vi "Do.vi"(8 "error in (no error)":errorcluster, 10 "Actor in":refnum<class "Actor.lvclass">, 11 "Execute Channel Msg":refnum<class "Execute Channel Msg.lvclass">) -> (0 "error out":errorcluster, 2 "Actor out":refnum<class "Actor.lvclass">)   [LabVIEW 2014, in "Generic Data Acquisition.lvlib" / "National Instrument USB-6501.lvlib" / "Execute Channel Msg.lvclass"]
doc: "This VI delivers the message to the actor by calling the appropriate method(s) on the actor."
uses:
  Execute Channel Msg.lvclass
  <vilib>/ActorFramework/Actor/Actor.lvclass
  National Instrument USB-6501/National Instrument USB-6501.lvclass
  Execute Channel Msg.lvclass/Execute Channel Msg.ctl
  <resource>/objmgr/daqmx.rc
panel:
  out "IsGlobal":bool
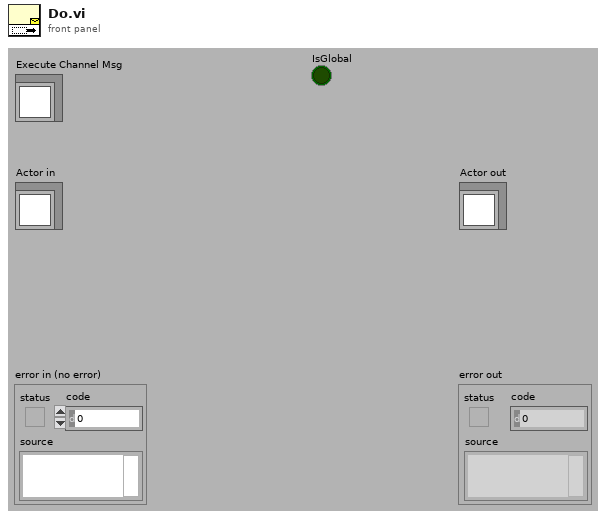
[diagram p1: front panel]
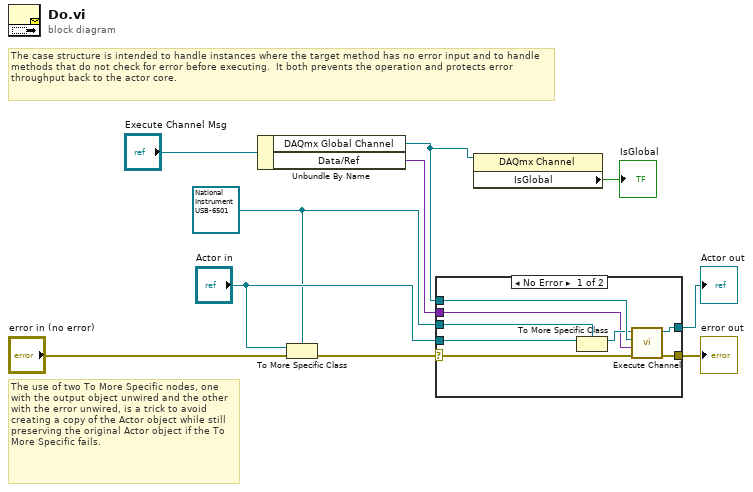
[diagram p0: block diagram]
diagram:
  w4 = refnum<class "National Instrument USB-6501.lvclass"> refnum ("Actor in")
  # "The use of two To More Specific nodes, one with the output object unwired and the other with the error unwired, is a trick to avoid creating a copy of the Actor object while still preserving the original Actor object if the To More Specific fails."
  # "The case structure is intended to handle instances where the target method has no error input and to handle methods that do not check for error before executing.  It both prevents the operation and protects error throughput back to the actor core."
  n1 = Unbundle By Name("Execute Channel Msg") -> ("DAQmx Global Channel"=w2:refnum<k21>, "Data/Ref"=w3:variant)
  n2 = To More Specific Class(target class=w4, reference="Actor in", error in="error in (no error)") -> (error out=w8:errorcluster)  [unwired: 1 out]
  n3 = case shown="No Error" w8 {
    selector: w8 -> [w16 w20]
    tunnel: [w18 w20] -> w7
    tunnel: [w17 w19] -> w6
    tunnel: "Actor in" -> [w15 w19]
    tunnel: w4 -> [w14 _]
    tunnel: w2 -> [w13 _]
    tunnel: w3 -> [w11 _]
    frame No Error {
      n4 = To More Specific Class(target class=w14, reference=w15) -> (specific class reference=w12:refnum<class "National Instrument USB-6501.lvclass">)  [unwired: 1 in, 1 out]
      n5 = call-dynamic "Execute Channel.vi"("error in (no error)"=w16, "Data/Ref"=w11, "DAQmx Global Channel"=w13, "National Instrument USB-6501 in"=w12) -> ("error out"=w18:errorcluster, "National Instrument USB-6501 out"=w17:refnum<class "National Instrument USB-6501.lvclass">)  [unwired: 6 in]
    }
    frame Error {
      # "If type check fails, pass the original object out again."
    }
  }
  "error out" <- w7
  "Actor out" <- w6
  n6 = property class="DAQmx Channel"(reference=w2) -> ("IsGlobal"=→"IsGlobal":bool)  [unwired: 1 in, 2 out]
